vi "Agilent 681x Acquire Power Measurement.vi"() -> ()   [LabVIEW 2019]
doc: "Shows how to acquire a power measurement using low level data VIs."
uses:
  <instrlib>/Agilent 681x Series/Public/Data/Low Level/Fetch Single Measurement (Power).vi
  <instrlib>/Agilent 681x Series/Agilent 681x Series.lvlib
panel:
  in  "Parar o programa":bool
  in  "Sample Spacing (25 us)":dbl=2.5e-05 format="%^.2g"
  in  "Sense Source (0: Internal)":u16(ring) items=["Internal", "External"]
  in  "Output Frequency (60 Hz)":dbl=60.0 format="%#.4g"
  in  "Voltage Amplitude (1.0 V)":dbl=1.0 format="%#.4g"
  in  "Relative Trigger Samples (0)":i32
  in  "Output Waveform Type (0: Sinusoid)":u16(ring) items=["Sinusoid", "Square", "Clipped Sinusoid", "User Specified"]
  out "Total Power":dbl
  out "Power Factor":dbl
  out "Reactive Power":dbl
  out "Apparent Power":dbl
  out "Real Power":dbl
  out "DC Power":dbl
  in  "Maximum Time (10000 ms)":i32=10000
  in  "User-Specified Output Waveform Name":string
  in  "Serial Configuration":T1={"Baud Rate"=9600, "Parity"=0, "Data Bits"=8} {"Data Bits" items=["7"=7, "8"=8]; "Parity" items=["None", "Odd", "Even", "Mark", "Space"]; "Baud Rate" items=["300"=300, "600"=600, "1200"=1200, "2400"=2400, "4800"=4800, "9600"=9600]}
  in  "VISA resource name":refnum<visa-resource-name>
  # "VI para definir:\n    1) amplitude da tensão de saída da fonte  (voltage amplitude)\n    2) fonte de medição (interna, externa) (sense source) e as especificações da medição (relative trigger samples, max time, sample spacing)"
  # "(c) 2008-2021 National Instruments Corp.  ALL RIGHTS RESERVED."
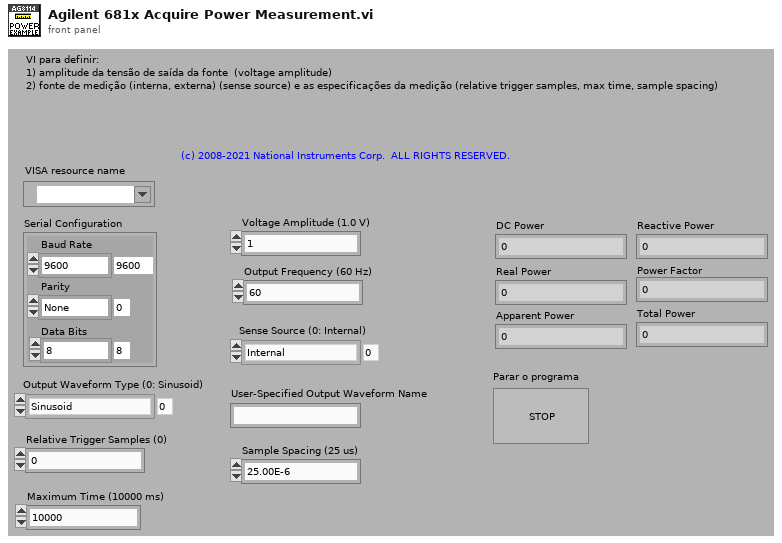
[diagram p1: front panel]
types:
  T1 = cluster{"Baud Rate":u32, "Parity":u16, "Data Bits":u16}
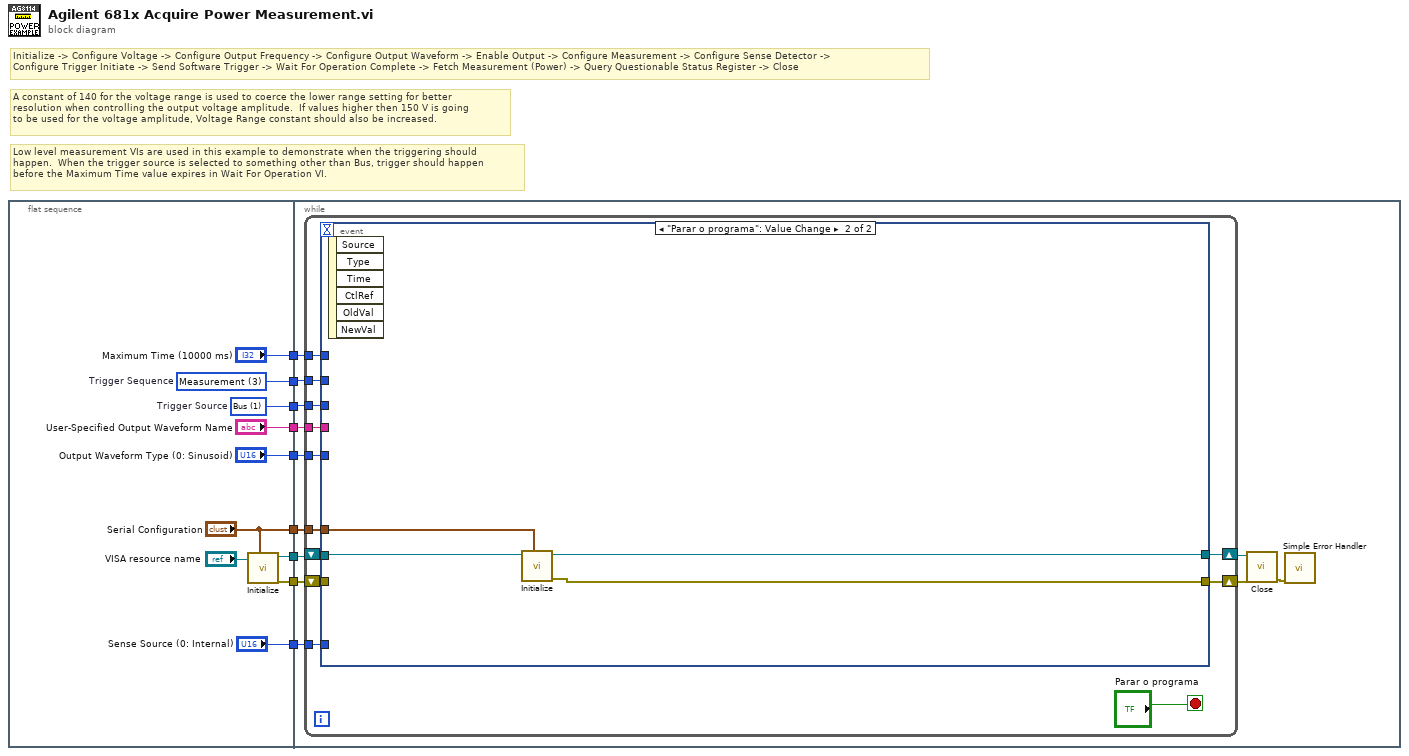
[diagram p0: block diagram]
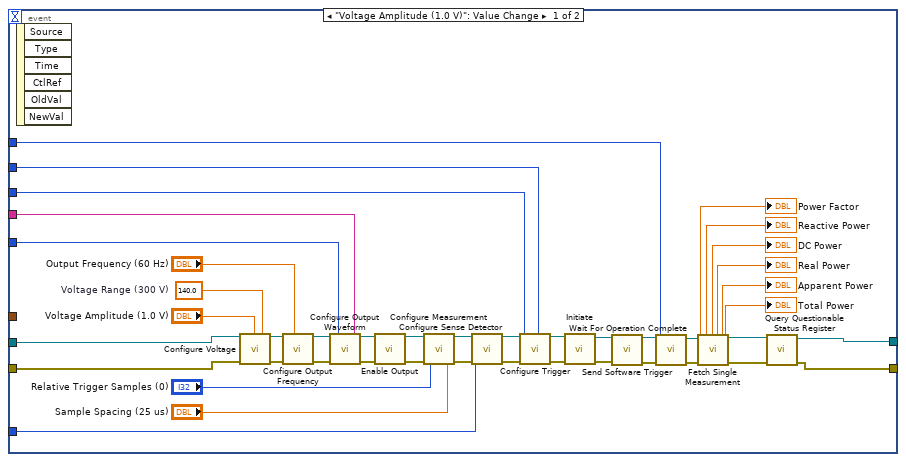
[diagram p2: hidden frame]
diagram:
  # "Initialize -> Configure Voltage -> Configure Output Frequency -> Configure Output Waveform -> Enable Output -> Configure Measurement -> Configure Sense Detector -> \nConfigure Trigger Initiate -> Send Software Trigger -> Wait For Operation Complete -> Fetch Measurement (Power) -> Query Questionable Status Register -> Close"
  # "Low level measurement VIs are used in this example to demonstrate when the triggering should\nhappen.  When the trigger source is selected to something other than Bus, trigger should happen\nbefore the Maximum Time value expires in Wait For Operation VI."
  # "A constant of 140 for the voltage range is used to coerce the lower range setting for better\nresolution when controlling the output voltage amplitude.  If values higher then 150 V is going\nto be used for the voltage amplitude, Voltage Range constant should also be increased."
  n1 = flat-sequence {
    tunnel: ["Maximum Time (10000 ms)"] -> w2
    tunnel: [w17] -> w3
    tunnel: [w16] -> w4
    tunnel: ["Sense Source (0: Internal)"] -> w5
    tunnel: ["User-Specified Output Waveform Name"] -> w6
    tunnel: ["Output Waveform Type (0: Sinusoid)"] -> w7
    tunnel: [w12] -> w8
    tunnel: [w11] -> w9
    tunnel: ["Serial Configuration"] -> w1
    tunnel: w9 -> [w24]
    tunnel: w8 -> [w25]
    tunnel: w7 -> [w26]
    tunnel: w6 -> [w27]
    tunnel: w5 -> [w28]
    tunnel: w4 -> [w29]
    tunnel: w3 -> [w30]
    tunnel: w2 -> [w31]
    tunnel: w1 -> [w21]
    frame #0 {
      w16 = 1 items=["Immediate", "Bus", "External", "Phase", "Trigger Out"]  # Trigger Source
      w17 = 3 items=["Output"=1, "Synchronous Source"=2, "Measurement"=3]  # Trigger Sequence
      n2 = call <instrlib>:"Initialize.vi"("Serial Configuration"="Serial Configuration", "VISA resource name"="VISA resource name") -> ("error out"=w11:errorcluster, "VISA resource name out"=w12:refnum<visa-resource-name>)  [unwired: 8 in]
    }
    frame #1 {
      n3 = while {
        tunnel: w31 -> [w43]
        tunnel: w30 -> [w42]
        tunnel: w29 -> [w41]
        tunnel: w28 -> [w40]
        tunnel: w27 -> [w39]
        tunnel: w26 -> [w38]
        shift-right: [w34] -> w22
        shift-left: w25 -> [w37]
        shift-right: [w35] -> w23
        shift-left: w24 -> [w36]
        tunnel: w21 -> [w33]
        stop <- "Parar o programa" stop-if-true
        n4 = event shown="[1] \"Parar o programa\": Value Change" {
          selector: _ -> [_ _]
          dyn-events: _ -> [_ _]
          timeout: _ -> [_ _]
          tunnel: w43 -> [w86 _]
          tunnel: w42 -> [w85 _]
          tunnel: w41 -> [w84 _]
          tunnel: w40 -> [w83 _]
          tunnel: w39 -> [w82 _]
          tunnel: w38 -> [w81 _]
          tunnel: w37 -> [w80 w89]
          tunnel: w36 -> [w79 _]
          tunnel: [w45 w87] -> w35
          tunnel: [w44 w88] -> w34
          tunnel: w33 -> [_ w90]
          event "Voltage Amplitude (1.0 V)": Value Change {
            w55 = 140.0  # Voltage Range (300 V)
            n5 = event-data() -> ()  [unwired: 1 in, 6 out]
            n6 = call <instrlib>:"Configure Voltage.vi"("VISA resource name"=w80, "Voltage Range (300 V)"=w55, "Voltage Amplitude (1.0 V)"="Voltage Amplitude (1.0 V)", "error in (no error)"=w79) -> ("VISA resource name out"=w66:refnum<visa-resource-name>, "error out"=w65:errorcluster)  [unwired: 10 in]
            n7 = call <instrlib>:"Configure Output Frequency.vi"("VISA resource name"=w66, "Output Frequency (60 Hz)"="Output Frequency (60 Hz)", "error in (no error)"=w65) -> ("VISA resource name out"=w60:refnum<visa-resource-name>, "error out"=w59:errorcluster)  [unwired: 11 in]
            n8 = call <instrlib>:"Configure Output Waveform.vi"("VISA resource name"=w60, "User-Specified Output Waveform Name"=w82, "Output Waveform Type (0: Sinusoid)"=w81, "error in (no error)"=w59) -> ("VISA resource name out"=w58:refnum<visa-resource-name>, "error out"=w57:errorcluster)  [unwired: 10 in]
            n9 = call <instrlib>:"Enable Output.vi"("VISA resource name"=w58, "error in (no error)"=w57) -> ("VISA resource name out"=w61:refnum<visa-resource-name>, "error out"=w62:errorcluster)  [unwired: 12 in]
            n10 = call <instrlib>:"Configure Measurement.vi"("VISA resource name"=w61, "Relative Trigger Samples (0)"="Relative Trigger Samples (0)", "Sample Spacing (25 us)"="Sample Spacing (25 us)", "error in (no error)"=w62) -> ("VISA resource name out"=w63:refnum<visa-resource-name>, "error out"=w64:errorcluster)  [unwired: 10 in]
            n11 = call <instrlib>:"Configure Sense Detector.vi"("VISA resource name"=w63, "Sense Source (0: Internal)"=w83, "error in (no error)"=w64) -> ("VISA resource name out"=w68:refnum<visa-resource-name>, "error out"=w67:errorcluster)  [unwired: 11 in]
            n12 = call <instrlib>:"Configure Trigger.vi"("VISA resource name"=w68, "Trigger Sequence (1: Output 1)"=w85, "Trigger Source (0: Immediate)"=w84, "error in (no error)"=w67) -> ("VISA resource name out"=w70:refnum<visa-resource-name>, "error out"=w69:errorcluster)  [unwired: 10 in]
            n13 = call <instrlib>:"Initiate.vi"("error in (no error)"=w69, "VISA resource name"=w70) -> ("error out"=w72:errorcluster, "VISA resource name out"=w71:refnum<visa-resource-name>)  [unwired: 8 in]
            n14 = call <instrlib>:"Send Software Trigger.vi"("VISA resource name"=w71, "error in (no error)"=w72) -> ("VISA resource name out"=w74:refnum<visa-resource-name>, "error out"=w73:errorcluster)  [unwired: 12 in]
            n15 = call <instrlib>:"Wait For Operation Complete.vi"("error in (no error)"=w73, "Maximum Time (10000 ms)"=w86, "VISA resource name"=w74) -> ("error out"=w76:errorcluster, "VISA resource name out"=w75:refnum<visa-resource-name>)  [unwired: 7 in]
            n16 = call-poly <instrlib>:"Fetch Single Measurement.vi"("VISA resource name"=w75, "error in (no error)"=w76) -> ("Power Factor"=→"Power Factor":dbl, "Reactive Power"=→"Reactive Power":dbl, "VISA resource name out"=w78:refnum<visa-resource-name>, "DC Power"=→"DC Power":dbl, "Real Power"=→"Real Power":dbl, "Apparent Power"=→"Apparent Power":dbl, "Total Power"=→"Total Power":dbl, "error out"=w77:errorcluster)  [unwired: 6 in]
            n17 = call <instrlib>:"Query Questionable Status Register.vi"("error in (no error)"=w77, "VISA resource name"=w78) -> ("error out"=w45:errorcluster, "VISA resource name out"=w44:refnum<visa-resource-name>)  [unwired: 7 in, 1 out]
          }
          event "Parar o programa": Value Change {
            n18 = event-data() -> ()  [unwired: 1 in, 6 out]
            n19 = call <instrlib>:"Initialize.vi"("Serial Configuration"=w90, "VISA resource name"=w89) -> ("error out"=w87:errorcluster, "VISA resource name out"=w88:refnum<visa-resource-name>)  [unwired: 8 in]
          }
        }
      }
      n20 = call <instrlib>:"Close.vi"("error in (no error)"=w23, "VISA resource name"=w22) -> ("error out"=w20:errorcluster)  [unwired: 9 in]
      n21 = call <vilib>:"Simple Error Handler.vi"("error in (no error)"=w20) -> ()  [unwired: 4 in, 5 out]
    }
  }
